vi "Created Events.vi"(8 "Created Event Alias":string, 9 "Priority?":bool, 10 "Msg Strategy":refnum<class "Msg Strategy.lvclass">, 11 "TEMPLATE Queue in":refnum<class "TEMPLATE Queue.lvclass">) -> (3 "TEMPLATE Queue out":refnum<class "TEMPLATE Queue.lvclass">)   [LabVIEW 2021, in "_Template.lvlib" / "Templates.lvlib" / "TEM Queue.lvlib" / "TEMPLATE Queue.lvclass"]
uses:
  TEMPLATE Queue.lvclass
  <vilib>/Nathan Davis/jettl/jettl/Msg Strategy/Msg Strategy.lvclass
  TEMPLATE Queue.lvclass/TEMPLATE Queue.ctl
  <vilib>/Nathan Davis/jettl/jettl/Queue/Queue.lvclass
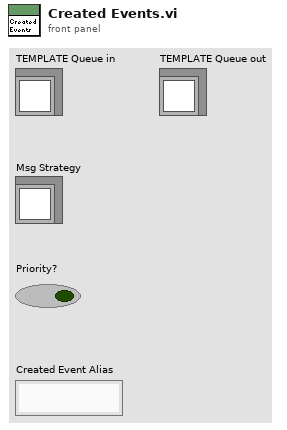
[diagram p1: front panel]
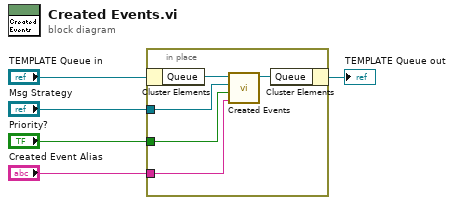
[diagram p0: block diagram]
diagram:
  n1 = in-place {
    in-place-border: "Msg Strategy" -> [w8]
    in-place-border: "Priority?" -> [w7]
    in-place-border: "Created Event Alias" -> [w6]
    n2 = in-place-cluster #1("TEMPLATE Queue in") -> ("Queue"=w10:refnum<class "Queue.lvclass">)
    n3 = call-dynamic "Created Events.vi"("Created Event Alias"=w6, "Priority?"=w7, "Msg Strategy"=w8, "Queue in"=w10) -> ("Queue out"=w9:refnum<class "Queue.lvclass">)  [unwired: 7 in]
    n4 = in-place-cluster #1("Queue"=w9) -> (→"TEMPLATE Queue out":refnum<class "TEMPLATE Queue.lvclass">)
  }
